vi "readLasers.vi"(5 "Prior Lows":u8=10, 6 "Laser Readings In":T1, 7 "Reset Count":bool, 8 "Simple Laser 2":bool, 9 "Simple Laser 1":bool, 10 "Fancy Laser 2":bool, 11 "Fancy Laser 1":bool) -> (4 "Laser Readings Out":T1)   [LabVIEW 2017]
uses:
  Downloads/Guadaloop-Pod-myRIO-System-Jaidev_v9-20180210T022027Z-001/Guadaloop-Pod-myRIO-System-Jaidev_v9/Guadaloop-Pod-myRIO-System-Jaidev_v9/Type Defs/allLaserReadings.ctl
  TypeDefs/laserReading.ctl
panel:
  # "default - 10"
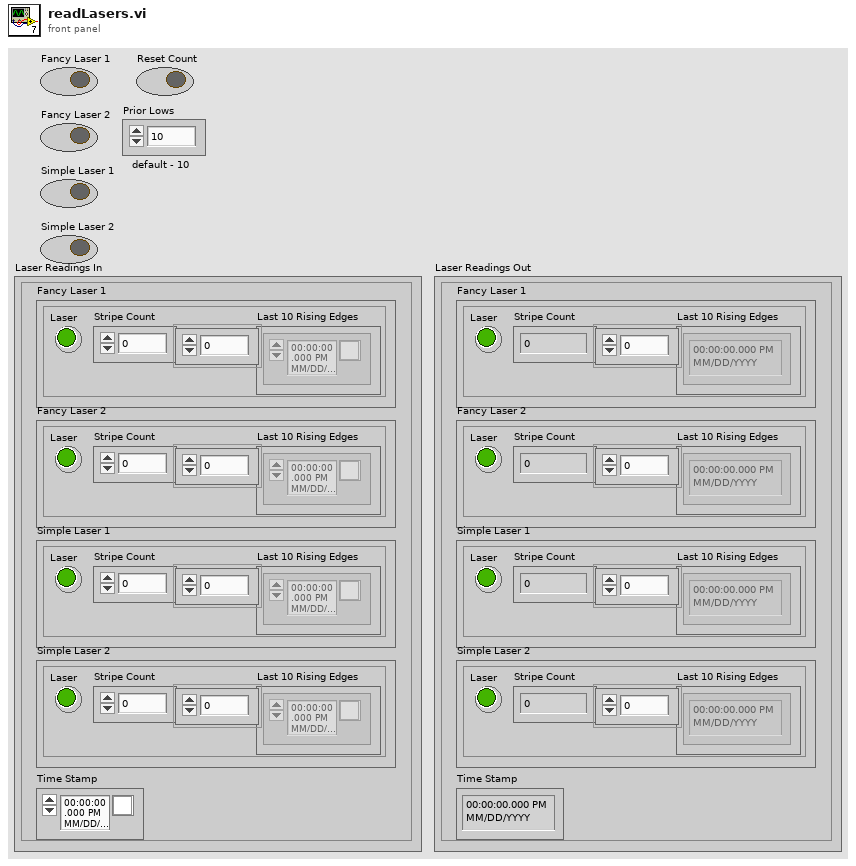
[diagram p1: front panel]
types:
  T1 = typedef "allLaserReadings.ctl" = cluster{"Fancy Laser 1":T2, "Fancy Laser 2":T2, "Simple Laser 1":T2, "Simple Laser 2":T2, "Time Stamp":timestamp}
  T2 = typedef "laserReading.ctl" = cluster{"Laser":bool, "Stripe Count":u32, "Last 10 Rising Edges":timestamp[]}
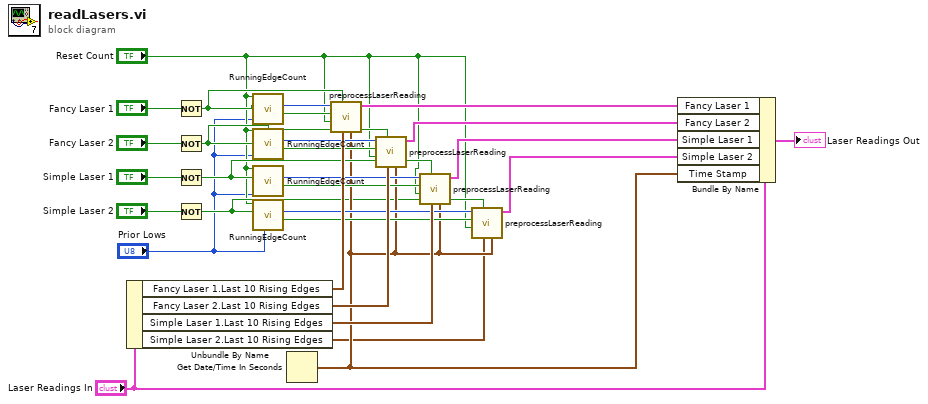
[diagram p0: block diagram]
diagram:
  n1 = Unbundle By Name("Laser Readings In") -> ("Fancy Laser 1.Last 10 Rising Edges"=w20:timestamp[], "Fancy Laser 2.Last 10 Rising Edges"=w16:timestamp[], "Simple Laser 1.Last 10 Rising Edges"=w13:timestamp[], "Simple Laser 2.Last 10 Rising Edges"=w4:timestamp[])
  n2 = Not(x="Fancy Laser 1") -> (.not. x?=w23:bool)
  n3 = Not(x="Fancy Laser 2") -> (.not. x?=w17:bool)
  n4 = Not(x="Simple Laser 1") -> (.not. x?=w12:bool)
  n5 = Not(x="Simple Laser 2") -> (.not. x?=w3:bool)
  n6 = call "RunningEdgeCount.vi"("Prior Lows"="Prior Lows", "Reset Count? (F)"="Reset Count", "Input"=w23) -> ("Rising Edge?"=w24:bool, "Count"=w25:u32)  [unwired: 7 in]
  n7 = call "RunningEdgeCount.vi"("Prior Lows"="Prior Lows", "Reset Count? (F)"="Reset Count", "Input"=w17) -> ("Rising Edge?"=w18:bool, "Count"=w19:u32)  [unwired: 7 in]
  n8 = call "RunningEdgeCount.vi"("Prior Lows"="Prior Lows", "Reset Count? (F)"="Reset Count", "Input"=w12) -> ("Rising Edge?"=w14:bool, "Count"=w15:u32)  [unwired: 7 in]
  n9 = call "RunningEdgeCount.vi"("Prior Lows"="Prior Lows", "Reset Count? (F)"="Reset Count", "Input"=w3) -> ("Rising Edge?"=w10:bool, "Count"=w11:u32)  [unwired: 7 in]
  n10 = Get Date/Time In Seconds() -> (seconds since 1Jan1904=w5:timestamp)
  n11 = call "preprocessLaserReading.vi"("Right Now"=w5, "Last 10 Rising Edges"=w20, "Laser On?"=w23, "Reset"="Reset Count", "Rising Edge?"=w24, "Count"=w25) -> ("Laser Reading"=w22:T2)  [unwired: 5 in]
  n12 = call "preprocessLaserReading.vi"("Right Now"=w5, "Last 10 Rising Edges"=w16, "Laser On?"=w17, "Reset"="Reset Count", "Rising Edge?"=w18, "Count"=w19) -> ("Laser Reading"=w9:T2)  [unwired: 5 in]
  n13 = call "preprocessLaserReading.vi"("Right Now"=w5, "Last 10 Rising Edges"=w13, "Laser On?"=w12, "Reset"="Reset Count", "Rising Edge?"=w14, "Count"=w15) -> ("Laser Reading"=w8:T2)  [unwired: 5 in]
  n14 = call "preprocessLaserReading.vi"("Right Now"=w5, "Last 10 Rising Edges"=w4, "Laser On?"=w3, "Reset"="Reset Count", "Rising Edge?"=w10, "Count"=w11) -> ("Laser Reading"=w7:T2)  [unwired: 5 in]
  n15 = Bundle By Name(cluster="Laser Readings In", "Fancy Laser 1"=w22, "Fancy Laser 2"=w9, "Simple Laser 1"=w8, "Simple Laser 2"=w7, "Time Stamp"=w5) -> (→"Laser Readings Out":T1)
